vi "Asylum_Driver_LowerTip.vi"(8 "error in (no error)":errorcluster, 10 "Z Setpoint":dbl, 11 "Application":refnum<k7>) -> (0 "error out":errorcluster, 3 "Application":refnum<k7>)   [LabVIEW 2019]
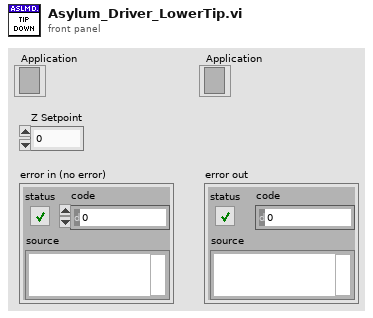
[diagram p1: front panel]
types:
  T1 = cluster{"setpoint":dbl, "pgain":dbl, "igain":dbl, "sgain":dbl}
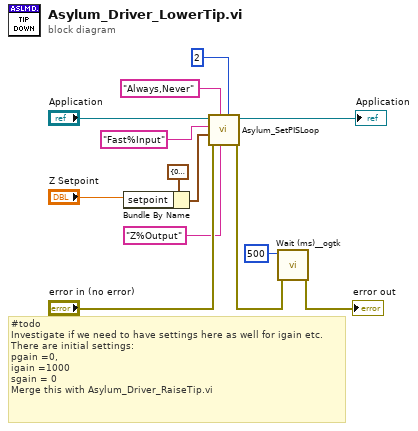
[diagram p0: block diagram]
diagram:
  # "#todo \nInvestigate if we need to have settings here as well for igain etc.\nThere are initial settings:\npgain =0,\nigain =1000\nsgain = 0\nMerge this with Asylum_Driver_RaiseTip.vi"
  n1 = Bundle By Name(cluster=T1 {"setpoint"=0.0, "pgain"=0.0, "igain"=1000.0, "sgain"=0.0} ("PIS Controls"), "setpoint"="Z Setpoint") -> (w2:T1)
  n2 = call <userlib>:"Asylum_SetPISLoop.vi"("whichLoop"=2, "outChannelString"="Z%Output", "eventString"="Always,Never", "error in (no error)"="error in (no error)", "PIS Controls"=w2, "inChannelString"="Fast%Input", "Application"="Application") -> ("error out"=w6:errorcluster, "Application"=→"Application":refnum<k7>)  [unwired: 3 in]
  n3 = call <userlib>:"Wait (ms)__ogtk.vi"("error in (no error)"=w6, "milliseconds to wait"=u32 500) -> ("error out"=→"error out":errorcluster)  [unwired: 8 in, 1 out]
